vi "Plot Spectrum.vi"(8 "error in (no error)":errorcluster, 10 "Channel":u8, 11 "Micron Optics Recorder in":refnum<class "Micron Optics Recorder.lvclass">) -> (0 "error out":errorcluster, 3 "Micron Optics Recorder out":refnum<class "Micron Optics Recorder.lvclass">)   [LabVIEW 2016, in "Micron Optics Recorder.lvclass"]
uses:
  Micron Optics Recorder.lvclass
  C:/github/LabActor/Template Module/Template Module.lvclass
  Template Module/Template Module.lvclass/Template Module.ctl
  Micron Optics Recorder.lvclass/Micron Optics Recorder.ctl
  Template Module/Read Configuration.vi
  NHMFL_Core/Libraries/Instruments/Micron Optics/Micron Optics Driver/Micron Optics Driver.lvclass
  C:/github/NHMFL_Core/Libraries/Instruments/Instrument Driver/Instrument Driver.lvclass
  Read Micron Optics Driver.vi
  NHMFL_Core/Libraries/Instruments/Instrument Driver/Write User configuration.vi
  Write Micron Optics Driver.vi
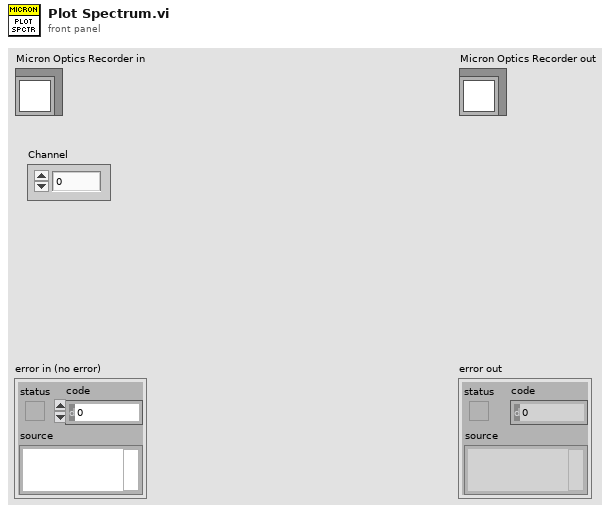
[diagram p1: front panel]
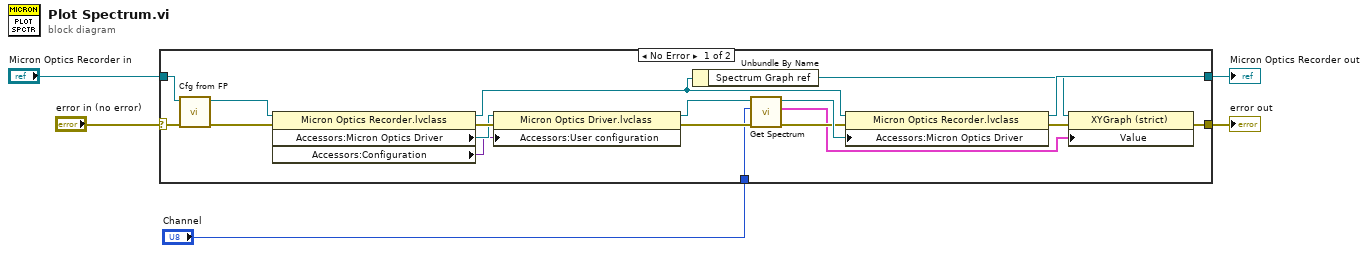
[diagram p0: block diagram]
diagram:
  n1 = case shown="No Error" "error in (no error)" {
    selector: "error in (no error)" -> [w13 w25]
    tunnel: [w17 w25] -> w4
    tunnel: [w21 w24] -> w2
    tunnel: "Micron Optics Recorder in" -> [w14 w24]
    tunnel: "Channel" -> [w6 _]
    frame No Error {
      n2 = call-dynamic "Cfg from FP.vi"("error in (no error)"=w13, "Measure Object in"=w14) -> ("error out"=w12:errorcluster, "Measure Object out"=w11:refnum<class "Micron Optics Recorder.lvclass">)  [unwired: 8 in]
      n3 = property class="Micron Optics Recorder.lvclass"(reference=w11, error in=w12) -> (reference out=w18:refnum<class "Micron Optics Recorder.lvclass">, error out=w23:errorcluster, "Accessors:Micron Optics Driver"=w9:refnum<class "Micron Optics Driver.lvclass">, "Accessors:Configuration"=w7:variant)
      n4 = property class="Micron Optics Driver.lvclass"(reference=w9, error in=w23, "Accessors:User configuration"=w7) -> (reference out=w8:refnum<class "Micron Optics Driver.lvclass">, error out=w10:errorcluster)
      n5 = Unbundle By Name(w18) -> ("Spectrum Graph ref"=w16:refnum<vi>)
      n6 = call-dynamic "Get Spectrum.vi"("error in (no error)"=w10, "Channel"=w6, "Micron Optics Driver in"=w8) -> ("error out"=w19:errorcluster, "Spectrum Graph"=w15:cluster{dbl[], "Spectrum, db":dbl[]}[], "Micron Optics Driver out"=w20:refnum<class "Micron Optics Driver.lvclass">)  [unwired: 6 in]
      n7 = property class="Micron Optics Recorder.lvclass"(reference=w18, error in=w19, "Accessors:Micron Optics Driver"=w20) -> (reference out=w21:refnum<class "Micron Optics Recorder.lvclass">, error out=w22:errorcluster)
      n8 = property class="XYGraph (strict)"(reference=w16, error in=w22, "Value"=w15) -> (error out=w17:errorcluster)  [unwired: 1 out]
    }
    frame Error {
    }
  }
  "error out" <- w4
  "Micron Optics Recorder out" <- w2
